vi "result.To JSON Tree.vi"(8 "error in (no error)":errorcluster, 11 "result in":refnum<class "result.lvclass">) -> (0 "error out":errorcluster, 2 "JSON out":refnum<class "JSON Null.lvclass">, 3 "result out":refnum<class "result.lvclass">)   [LabVIEW 2016, in "result.lvclass"]
uses:
  result.lvclass
  <vilib>/NI/JSON Support for LabVIEW/JSON Data Classes/JSON Datatype/JSON Null.lvclass
  result.lvclass/result.ctl
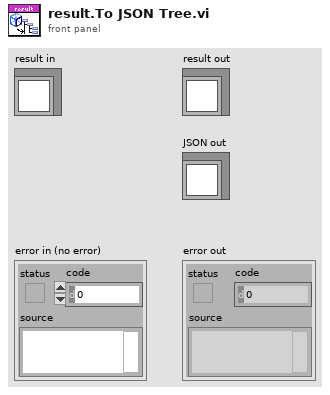
[diagram p1: front panel]
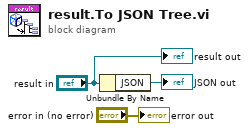
[diagram p0: block diagram]
diagram:
  n1 = Unbundle By Name("result in") -> ("JSON"=→"JSON out":refnum<class "JSON Null.lvclass">)
  "error out" <- "error in (no error)"
  "result out" <- "result in"
